vi "Update sim globals from JSON protocol.vi"(10 "Initialize":bool, 11 "Data":string) -> (1 "SimDevice":bool)   [LabVIEW 2020]
uses:
  <vilib>/Rock Robotics/WPI/Simulation/Protocol/Devices/Accel/Accel Update Ops.ctl
  <vilib>/Rock Robotics/WPI/Simulation/Protocol/Devices/AI/AI Update Ops.ctl
  <vilib>/Rock Robotics/WPI/Simulation/Protocol/Devices/AO/AO Update Ops.ctl
  <vilib>/Rock Robotics/WPI/Simulation/Protocol/Devices/DIO/DIO Update Ops.ctl
  <vilib>/Rock Robotics/WPI/Simulation/Protocol/Devices/dPWM/dPWM Update Ops.ctl
  <vilib>/Rock Robotics/WPI/Simulation/Protocol/Devices/DriverStation/DS Update Ops.ctl
  <vilib>/Rock Robotics/WPI/Simulation/Protocol/Devices/DutyCycle/DutyCycle Update Ops.ctl
  <vilib>/Rock Robotics/WPI/Simulation/Protocol/Devices/Encoder/Encoder Update Ops.ctl
  Devices/Gyro/Gyro Update Ops.ctl
  <vilib>/Rock Robotics/WPI/Simulation/Protocol/Devices/Joystick/Joystick Update Ops.ctl
  <vilib>/Rock Robotics/WPI/Simulation/Protocol/Devices/PWM/PWM Update Ops.ctl
  <vilib>/Rock Robotics/WPI/Simulation/Protocol/Devices/Relay/Relay Update Ops.ctl
  <vilib>/Rock Robotics/WPI/Simulation/Protocol/Devices/RoboRIO/RoboRIO Update Ops.ctl
  Devices/RomiGyro/RomiGyro Update Ops.ctl
  Devices/CTREPCM/CTREPCM Update Ops.ctl
  Devices/Solenoid/Solenoid Update Ops.ctl
  <vilib>/MultiError/TokenizeJSON/Multi Error Cluster.lvlib
  <vilib>/Utility/Data Type/NI_Data Type.lvlib
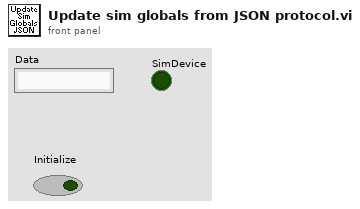
[diagram p1: front panel]
types:
  T1 = cluster{string[], refnum<vi>[], cluster{"index of element":i32, "index of element":i32}[]}
  T2 = cluster{"index of element":i32, "index of element":i32}
  T3 = typedef "Multi Error Cluster.lvlib/JSON Token Descriptor.ctl" = cluster{"match string":string, "raw token type":T4, "byte offset ":i32}
  T4 = typedef "Multi Error Cluster.lvlib/JSON Raw Token Values.ctl" = enum32{"{", "}", "[", "]", ",", ":", "\"", "number", "string", "true", "false", "null", "invalid"}
  T5 = typedef "Multi Error Cluster.lvlib/JSON Token Values.ctl" = enum32{"array begin", "array end", "object begin", "object end", "value", "invalid", "name"}
  T6 = cluster{"whole match":string, "token index":i32}[]
  T7 = typedef "Accel Update Ops.ctl" = enum16{"get", "delete", "JSON update", "set  name", "transmit initial", "reset", "set init", "set range"}
  T8 = typedef "AI Update Ops.ctl" = enum16{"set init", "set avg_bits", "set oversample_bits", "set voltage", "set Accum_init", "set Accum_value", "set Accum_count", "set Accum_center", "set Accum_deadband", "get", "delete", "JSON update", "set  name", "transmit initial", "reset"}
  T9 = typedef "AO Update Ops.ctl" = enum16{"set init", "set value", "JSON update", "set name", "transmit initial", "get", "delete", "reset"}
  T10 = typedef "DIO Update Ops.ctl" = enum16{"set init", "set value", "set pulse_length", "set input", "get", "delete", "JSON update", "set name", "transmit initial", "reset"}
  T11 = typedef "dPWM Update Ops.ctl" = enum16{"get", "delete", "JSON update", "set  name", "transmit initial", "reset", "set init", "set duty cycle", "set dio channel"}
  T12 = typedef "DS Update Ops.ctl" = enum16{"set enabled", "set autonomous", "set test", "set estop", "set fms", "set ds", "set control word", "set match_time", "set station", "set game data", "JSON update", "set name", "get", "transmit initial", "reset"}
  T13 = typedef "DutyCycle Update Ops.ctl" = enum16{"get", "delete", "JSON update", "set  name", "transmit initial", "reset", "set init"}
  T14 = typedef "Encoder Update Ops.ctl" = enum16{"set init", "set count", "set period", "set reset", "set samples_to_avg", "get", "delete", "JSON update", "set name", "transmit initial", "reset", "set channel_a", "set channel_b"}
  T15 = typedef "Gyro Update Ops.ctl" = enum16{"get", "delete", "JSON update", "set  name", "transmit initial", "reset", "set init", "set offsetX", "set offsetY", "set offsetZ", "set gain", "set angle X", "set angle Y", "set angle Z", "set rate X", "set rate Y", "set rate Z"}
  T16 = typedef "Joystick Update Ops.ctl" = enum16{"set init", "set buttons", "set povs", "set axes", "set left_rumble", "set right_rumble", "set outputs", "get", "delete", "JSON update", "set name", "transmit initial", "reset"}
  T17 = typedef "PWM Update Ops.ctl" = enum16{"set init", "set speed", "set position", "set raw", "set  period_scale", "set zero_latch", "set angular range", "get", "delete", "JSON update", "set name", "transmit initial", "reset"}
  T18 = typedef "Relay Update Ops.ctl" = enum16{"set init_fwd", "set init_rev", "set fwd", "set rev", "get", "delete", "JSON update", "set name", "transmit initial", "reset"}
  T19 = typedef "RoboRIO Update Ops.ctl" = enum16{"get", "JSON update", "set name", "transmit initial", "set fpga_button", "set vin_voltage", "set vin_current", "set 6v_voltage", "set 6v_current", "set 6v_active", "set 6v_faults", "set 5v_voltage", "set 5v_current", "set 5v_active", "set 5v_faults", "set 3v3_voltage", "set 3v3_current", "set 3v3_active", "set 3v3_faults", "reset"}
  T20 = typedef "RomiGyro Update Ops.ctl" = enum16{"get", "delete", "JSON update", "set  name", "transmit initial", "reset", "set init", "set rate_x", "set rate_y", "set rate_z", "set angle_x", "set angle_y", "set angle_z", "set offset_x", "set offset_y", "set offset_z"}
  T21 = typedef "CTREPCM Update Ops.ctl" = enum16{"get", "delete", "JSON update", "set  name", "transmit initial", "reset", "set init", "set compressor on", "set closed loop", "set pressure switch", "set current"}
  T22 = typedef "Solenoid Update Ops.ctl" = enum16{"get", "delete", "JSON update", "set  name", "transmit initial", "reset", "set init", "set output"}
  T23 = cluster{"index of element":i32, "index of element":i32}[]
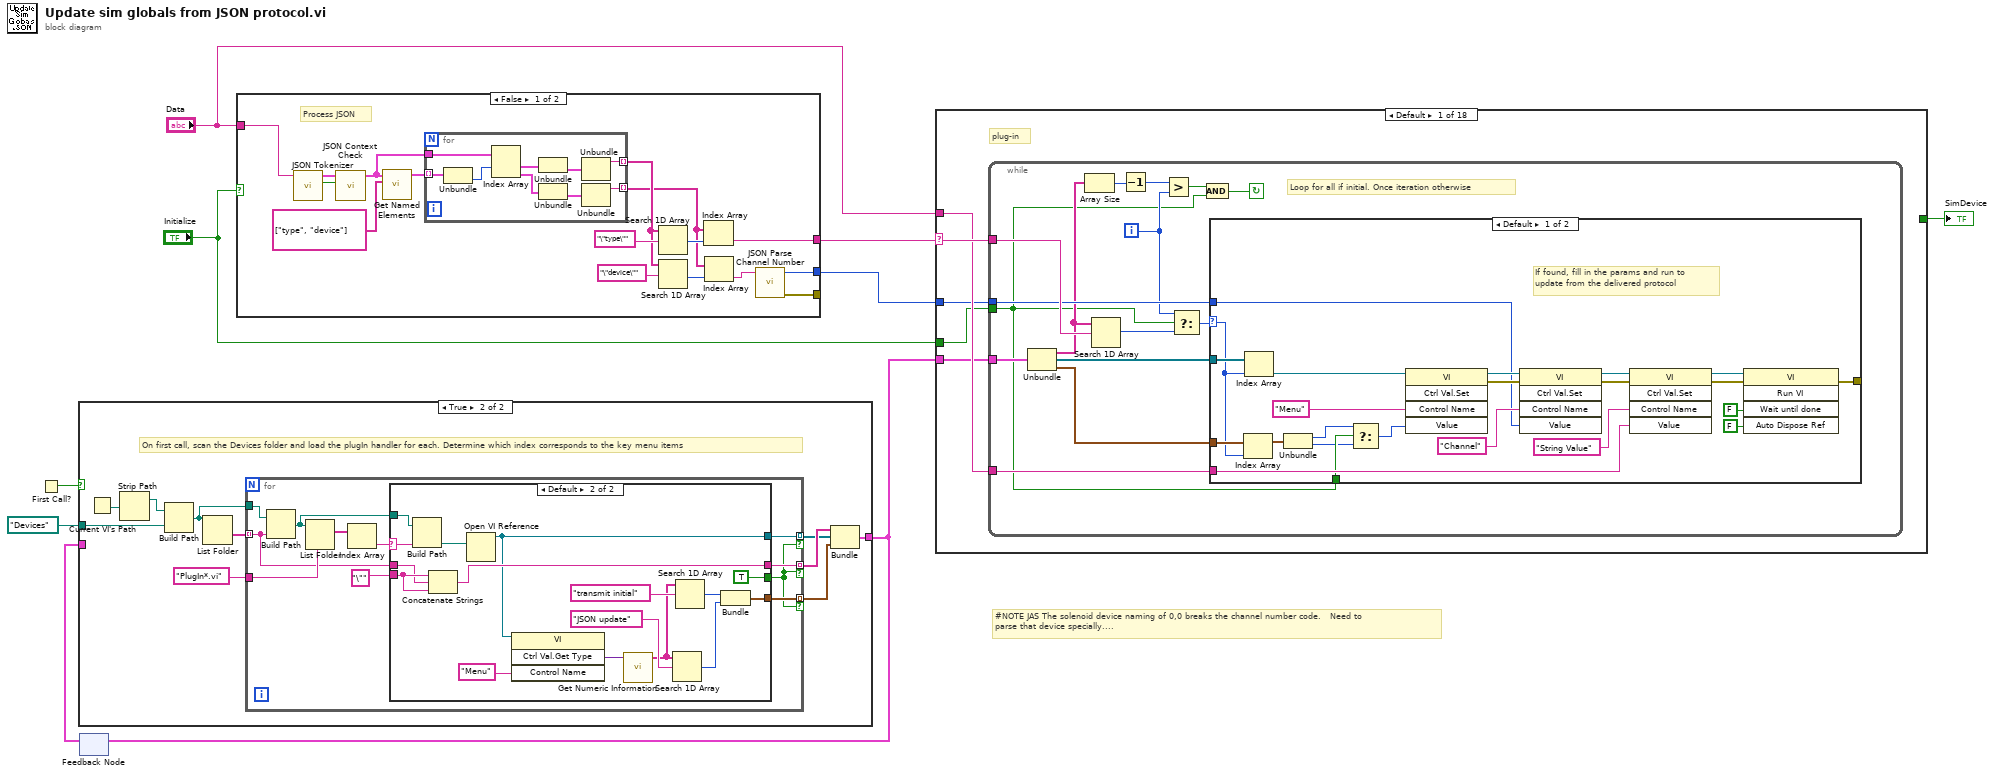
[diagram p0: block diagram]
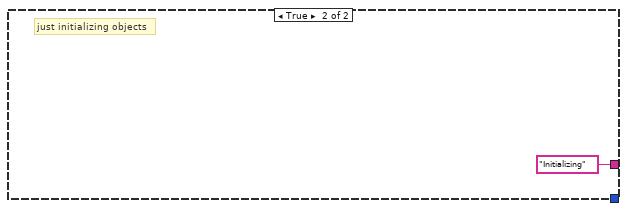
[diagram p2: hidden frame]
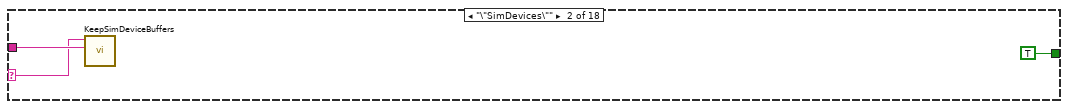
[diagram p6: hidden frame]
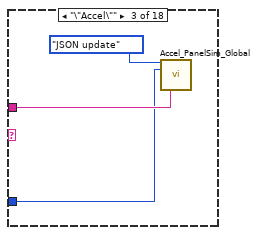
[diagram p7: hidden frame]
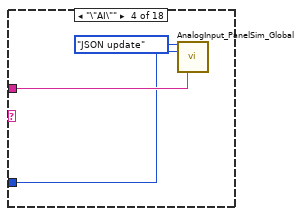
[diagram p8: hidden frame]
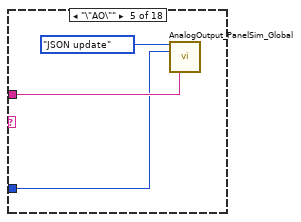
[diagram p9: hidden frame]
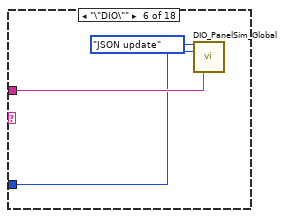
[diagram p10: hidden frame]
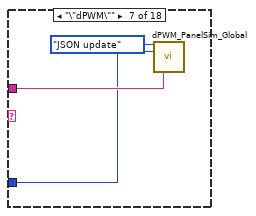
[diagram p11: hidden frame]
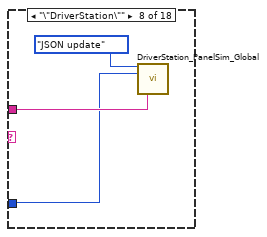
[diagram p12: hidden frame]
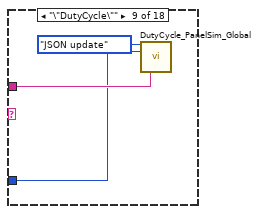
[diagram p13: hidden frame]
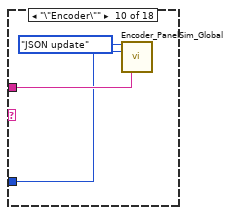
[diagram p14: hidden frame]
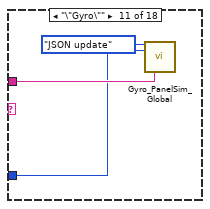
[diagram p15: hidden frame]
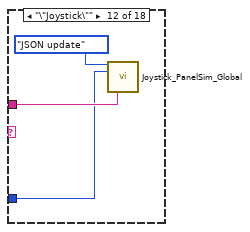
[diagram p16: hidden frame]
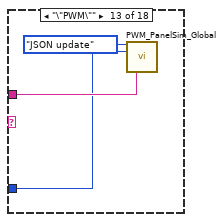
[diagram p17: hidden frame]
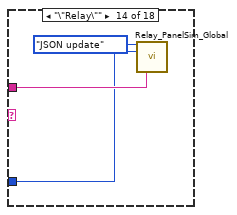
[diagram p18: hidden frame]
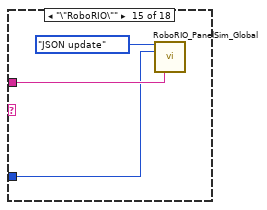
[diagram p19: hidden frame]
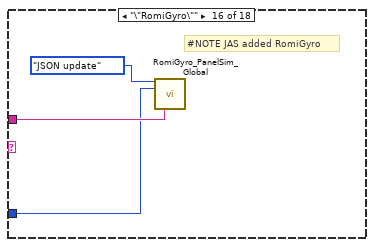
[diagram p20: hidden frame]
diagram:
  # "#NOTE JAS The solenoid device naming of 0,0 breaks the channel number code.   Need to\nparse that device specially...."
  n1 = First Call?() -> (First Call?: T/F=w6:bool)
  n2 = feedback #1() -> (w4:T1)  [unwired: 1 in]
  n3 = case shown="True" w6 {
    tunnel: path "Devices" -> [_ w20]
    tunnel: [w10 w12] -> w2
    tunnel: w4 -> [w10 _]
    frame False {
    }
    frame True {
      # "On first call, scan the Devices folder and load the plugIn handler for each. Determine which index corresponds to the key menu items"
      n4 = Current VI's Path() -> (path=w19:path)
      n5 = Strip Path(path=w19) -> (stripped path=w18:path)  [unwired: 1 out]
      n6 = Build Path(base path=w18, name or relative path=w20) -> (appended path=w16:path)
      n7 = List Folder(path=w16) -> (folder names=w17:string[])  [unwired: 3 in, 3 out]
      n8 = for {
        tunnel: w17 -> [w27] mode=indexing
        tunnel: w16 -> [w31]
        tunnel: "PlugIn*.vi" ("pattern") -> [w30]
        tunnel: [w26] -> w13 mode=indexing if=w21
        tunnel: [w25] -> w14 mode=indexing if=w21
        tunnel: [w22] -> w11 mode=indexing if=w21
        n9 = Build Path(base path=w31, name or relative path=w27) -> (appended path=w24:path)
        n10 = List Folder(path=w24, pattern=w30) -> (filenames=w29:string[])  [unwired: 2 in, 3 out]
        n11 = Index Array(array=w29) -> (element=w28:string)  [unwired: 1 in]
        n12 = case shown="Default" w28 {
          selector: w28 -> [_ w46]
          tunnel: [_ w39] -> w26
          tunnel: w27 -> [_ w41]
          tunnel: [_ w42] -> w25
          tunnel: [_ TRUE] -> w21
          tunnel: w24 -> [_ w45]
          tunnel: "\"" -> [_ w43]
          tunnel: [_ w32] -> w22
          frame "", "Tmpl_PanelSim_Global.vi" {
            # "not found\nor tmpl"
          }
          frame Default {
            n13 = Build Path(base path=w45, name or relative path=w46) -> (appended path=w44:path)
            n14 = Concatenate Strings(w43, w41, w43) -> (w42:string)
            n15 = Open VI Reference(vi path=w44) -> (vi reference=w39:refnum<vi>)  [unwired: 5 in, 1 out]
            n16 = invoke class="VI" method="Ctrl Val.Get Type"(reference=w39, "Control Name"="Menu" ("whole match")) -> ("Ctrl Val.Get Type"=w40:variant)  [unwired: 2 in, 3 out]
            n17 = call <vilib>:"Get Numeric Information.vi"("variant"=w40) -> ("enum names"=w35:string[])  [unwired: 7 in, 3 out]
            n18 = Search 1D Array(1D array=w35, element="JSON update" ("whole match")) -> (index of element=w33:i32)  [unwired: 1 in]
            n19 = Search 1D Array(1D array=w35, element="transmit initial" ("whole match")) -> (index of element=w34:i32)  [unwired: 1 in]
            n20 = Bundle("index of element"=w34, "index of element"=w33) -> (w32:T2)  [unwired: 1 in]
          }
        }
      }
      n21 = Bundle(w14, w13, w11) -> (w12:T1)  [unwired: 1 in]
    }
  }
  n22 = feedback-in #1(w2) -> ()
  n23 = case shown="False" "Initialize" {
    tunnel: [w63 "Initializing" ("whole match")] -> w9
    tunnel: "Data" -> [w62 _]
    tunnel: [w49 _] -> w8
    tunnel: [w48 _] -> _
    frame False {
      # "Process JSON"
      n24 = call <vilib>:"JSON Tokenizer.vi"("JSON String"=w62) -> ("Invalid"=w56:bool, "Array"=w55:T3[])  [unwired: 9 in]
      n25 = call <vilib>:"JSON Context Check.vi"("Invalid in"=w56, "Parse Tokens in"=w55) -> ("tokens"=w60:cluster{"token type":T5, T3}[])  [unwired: 8 in, 1 out]
      n26 = call <vilib>:"Get Named Elements.vi"("names"=string[] ["type", "device"], "tokens"=w60) -> ("Found Token Info"=w57:T6)  [unwired: 9 in]
      n27 = for {
        tunnel: w57 -> [w72] mode=indexing
        tunnel: w60 -> [w71]
        tunnel: [w67] -> w53 mode=indexing
        tunnel: [w64] -> w52 mode=indexing
        n28 = Unbundle(w72) -> ("token index"=w70:i32)  [unwired: 1 out]
        n29 = Index Array(array=w71, index #1=w70) -> (element #1=w69:cluster{"token type":T5, T3}, element #2=w65:cluster{"token type":T5, T3})  [unwired: 1 in]
        n30 = Unbundle(w69) -> (w68:T3)  [unwired: 1 out]
        n31 = Unbundle(w65) -> (w66:T3)  [unwired: 1 out]
        n32 = Unbundle(w68) -> ("match string"=w67:string)  [unwired: 2 out]
        n33 = Unbundle(w66) -> ("match string"=w64:string)  [unwired: 2 out]
      }
      n34 = Search 1D Array(1D array=w53, element="\"type\"" ("whole match")) -> (index of element=w59:i32)  [unwired: 1 in]
      n35 = Search 1D Array(1D array=w53, element="\"device\"" ("whole match")) -> (index of element=w51:i32)  [unwired: 1 in]
      n36 = Index Array(array=w52, index=w59) -> (element=w63:string)
      n37 = Index Array(array=w52, index=w51) -> (element=w50:string)
      n38 = call "JSON Parse Channel Number.vi"("device string"=w50) -> ("error out"=w48:errorcluster, "Channel"=w49:i32)  [unwired: 9 in]
    }
    frame True {
      # "just initializing objects"
    }
  }
  n39 = case shown="Default" w9 {
    selector: w9 -> [w78 w118 _ _ _ _ _ _ _ _ _ _ _ _ _ _ _ _]
    tunnel: "Data" -> [w77 w119 w122 w125 w128 w131 w134 w137 w140 w143 w146 w149 w152 w155 w158 w161 w164 w167]
    tunnel: w8 -> [w76 _ w120 w123 w127 w130 w133 w135 w139 w142 w145 w147 w151 w154 w157 w160 w163 w166]
    tunnel: [_ TRUE _ _ _ _ _ _ _ _ _ _ _ _ _ _ _ _] -> w7
    tunnel: w2 -> [w75 _ _ _ _ _ _ _ _ _ _ _ _ _ _ _ _ _]
    tunnel: "Initialize" -> [w74 _ _ _ _ _ _ _ _ _ _ _ _ _ _ _ _ _]
    frame Default {
      # "plug-in"
      n40 = while {
        tunnel: w78 -> [w93]
        tunnel: w77 -> [w92]
        tunnel: w76 -> [w91]
        tunnel: w75 -> [w90]
        tunnel: w74 -> [w79]
        i -> [w83]
        stop <- w80 continue-if-true
        # "Loop for all if initial. Once iteration otherwise"
        n41 = Unbundle(w90) -> (w85:string[], w89:refnum<vi>[], w86:T23)
        n42 = Array Size(array=w85) -> (size(s)=w84:i32)
        n43 = Search 1D Array(1D array=w85, element=w93) -> (index of element=w87:i32)  [unwired: 1 in]
        n44 = Decrement(x=w84) -> (x-1=w82:i32)
        n45 = Greater?(x=w82, y=w83) -> (0:w81:bool)
        n46 = Select(t=w83, s=w79, f=w87) -> (s? t:f=w88:i32)
        n47 = And(x=w81, y=w79) -> (x .and. y?=w80:bool)
        n48 = case shown="Default" w88 {
          selector: w88 -> [w100 _]
          tunnel: w89 -> [w116 _]
          tunnel: w92 -> [w110 _]
          tunnel: [w104 _] -> _
          tunnel: w86 -> [w101 _]
          tunnel: w79 -> [w98 _]
          tunnel: w91 -> [w94 _]
          frame Default {
            # "If found, fill in the params and run to\nupdate from the delivered protocol"
            n49 = Index Array(array=w101, index=w100) -> (element=w99:T2)
            n50 = Index Array(array=w116, index=w100) -> (element=w103:refnum<vi>)
            n51 = Unbundle(w99) -> ("index of element"=w97:i32, "index of element"=w96:i32)
            n52 = Select(t=w97, s=w98, f=w96) -> (s? t:f=w95:i32)
            n53 = invoke class="VI" method="Ctrl Val.Set"(reference=w103, "Control Name"="Menu" ("whole match"), "Value"=w95) -> (reference out=w115:refnum<vi>, error out=w107:errorcluster)  [unwired: 2 in, 3 out]
            n54 = invoke class="VI" method="Ctrl Val.Set"(reference=w115, error in=w107, "Control Name"="Channel" ("whole match"), "Value"=w94) -> (reference out=w114:refnum<vi>, error out=w106:errorcluster)  [unwired: 1 in, 3 out]
            n55 = invoke class="VI" method="Ctrl Val.Set"(reference=w114, error in=w106, "Control Name"="String Value" ("whole match"), "Value"=w110) -> (reference out=w113:refnum<vi>, error out=w105:errorcluster)  [unwired: 1 in, 3 out]
            n56 = invoke class="VI" method="Run VI"(reference=w113, error in=w105, "Wait until done"=FALSE ("Wait Until Done"), "Auto Dispose Ref"=FALSE ("Auto Dispose Reference")) -> (error out=w104:errorcluster)  [unwired: 1 in, 4 out]
          }
          frame -1 {
            # "not found"
          }
        }
      }
    }
    frame "\"SimDevices\"" {
      n57 = call <vilib>:"KeepSimDeviceBuffers.vi"("Bufer"=w119, "Type of device"=w118) -> ()  [unwired: 10 in]
    }
    frame "\"Accel\"" {
      n58 = call <vilib>:"Accel_PanelSim_Global.vi"("Menu"=Accel_Update_Ops."JSON update", "Channel"=w120, "String Value"=w122) -> ()  [unwired: 11 in, 2 out]
    }
    frame "\"AI\"" {
      n59 = call <vilib>:"AnalogInput_PanelSim_Global.vi"("menu"=AI_Update_Ops."JSON update", "Channel"=w123, "String Value"=w125) -> ()  [unwired: 11 in, 2 out]
    }
    frame "\"AO\"" {
      n60 = call <vilib>:"AnalogOutput_PanelSim_Global.vi"("menu"=AO_Update_Ops."JSON update", "AO Channel"=w127, "JSON"=w128) -> ()  [unwired: 11 in, 2 out]
    }
    frame "\"DIO\"" {
      n61 = call <vilib>:"DIO_PanelSim_Global.vi"("menu"=DIO_Update_Ops."JSON update", "DIO Channel"=w130, "String Value"=w131) -> ()  [unwired: 11 in, 2 out]
    }
    frame "\"dPWM\"" {
      n62 = call <vilib>:"dPWM_PanelSim_Global.vi"("Menu"=dPWM_Update_Ops."JSON update", "DIO Channel"=w133, "String Value"=w134) -> ()  [unwired: 11 in, 2 out]
    }
    frame "\"DriverStation\"" {
      n63 = call <vilib>:"DriverStation_PanelSim_Global.vi"("menu"=DS_Update_Ops."JSON update", "Channel"=w135, "String Value"=w137) -> ()  [unwired: 11 in, 2 out]
    }
    frame "\"DutyCycle\"" {
      n64 = call <vilib>:"DutyCycle_PanelSim_Global.vi"("Menu"=DutyCycle_Update_Ops."JSON update", "Channel"=w139, "String Value"=w140) -> ()  [unwired: 11 in, 2 out]
    }
    frame "\"Encoder\"" {
      n65 = call <vilib>:"Encoder_PanelSim_Global.vi"("menu"=Encoder_Update_Ops."JSON update", "EncoderIndex"=w142, "String Value"=w143) -> ()  [unwired: 11 in, 2 out]
    }
    frame "\"Gyro\"" {
      n66 = call "Gyro_PanelSim_Global.vi"("Menu"=Gyro_Update_Ops."JSON update", "Channel"=w145, "String Value"=w146) -> ()  [unwired: 11 in, 2 out]
    }
    frame "\"Joystick\"" {
      n67 = call <vilib>:"Joystick_PanelSim_Global.vi"("menu"=Joystick_Update_Ops."JSON update", "JoystickDevice"=w147, "String Value"=w149) -> ()  [unwired: 11 in, 2 out]
    }
    frame "\"PWM\"" {
      n68 = call <vilib>:"PWM_PanelSim_Global.vi"("menu"=PWM_Update_Ops."JSON update", "PWMChannel"=w151, "String Value"=w152) -> ()  [unwired: 11 in, 2 out]
    }
    frame "\"Relay\"" {
      n69 = call <vilib>:"Relay_PanelSim_Global.vi"("menu"=Relay_Update_Ops."JSON update", "RelayChannel"=w154, "String Value"=w155) -> ()  [unwired: 11 in, 2 out]
    }
    frame "\"RoboRIO\"" {
      n70 = call <vilib>:"RoboRIO_PanelSim_Global.vi"("Menu"=RoboRIO_Update_Ops."JSON update", "Channel"=w157, "String Value"=w158) -> ()  [unwired: 11 in, 2 out]
    }
    frame "\"RomiGyro\"" {
      # "#NOTE JAS added RomiGyro"
      n71 = call "RomiGyro_PanelSim_Global.vi"("Menu"=RomiGyro_Update_Ops."JSON update", "Channel"=w160, "String Value"=w161) -> ()  [unwired: 11 in, 2 out]
    }
    frame "\"CTREPCM\"" {
      # "#NOTE JAS added CTREPCM"
      n72 = call "CTREPCM_PanelSim_Global.vi"("Menu"=CTREPCM_Update_Ops."JSON update", "Channel"=w163, "String Value"=w164) -> ()  [unwired: 11 in, 2 out]
    }
    frame "\"Solenoid\"" {
      # "#NOTE JAS added Solenoid"
      n73 = call "Solenoid_PanelSim_Global.vi"("Menu"=Solenoid_Update_Ops."JSON update", "Channel"=w166, "String Value"=w167) -> ()  [unwired: 11 in, 2 out]
    }
  }
  "SimDevice" <- w7
